vi "get indices.vi"(7 "Category":string, 11 "array in":string[](array[string])) -> (3 "Indices":i32[](array[numeric]))   [LabVIEW 2013, in "PL Framework Configuration Tool.lvlib" / "Engine Parent Editor Node.lvclass"]
uses:
  Engine Parent Editor Node.lvclass
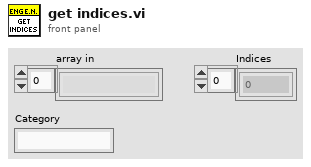
[diagram p1: front panel]
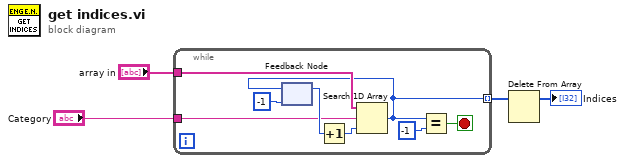
[diagram p0: block diagram]
diagram:
  n1 = while {
    tunnel: "array in" -> [w12]
    tunnel: [w6] -> w2 mode=indexing
    tunnel: "Category" -> [w5]
    stop <- w10 stop-if-true
    n2 = feedback #1(-1) -> (w7:i32)
    n3 = Increment(x=w7) -> (x+1=w8:i32)
    n4 = Search 1D Array(1D array=w12, element=w5, start index (0)=w8) -> (index of element=w6:i32)
    n5 = feedback-in #1(w6) -> ()
    n6 = Equal?(x=w6, y=-1) -> (x = y?=w10:bool)
  }
  n7 = Delete From Array(array=w2) -> (array with subset deleted=→"Indices":i32[])  [unwired: 2 in, 1 out]
